vi "Tell Parent Inspect.vi"(4 "Msg":refnum<class "Msg.lvclass">, 6 "Within Unified Msgs":bool, 7 "Actor in":refnum<class "Actor.lvclass">, 8 "Error in":errorcluster) -> (0 "Error out":errorcluster, 2 "Proceed":bool=TRUE, 5 "Actor out":refnum<class "Actor.lvclass">)   [LabVIEW 2025, in "jettl.lvlib"]
uses:
  jettl.lvlib
  Actor/Actor.lvclass
  Msg/Msg.lvclass
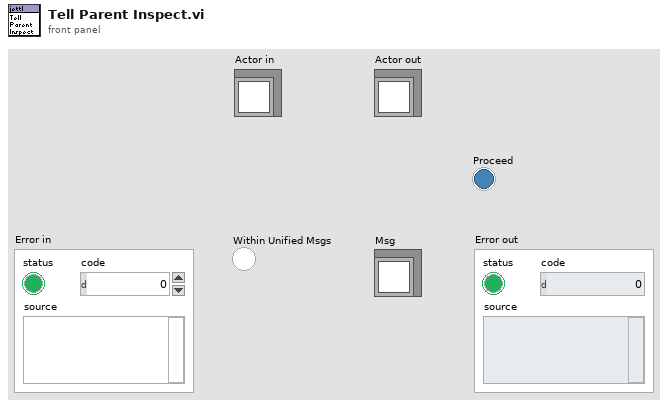
[diagram p1: front panel]
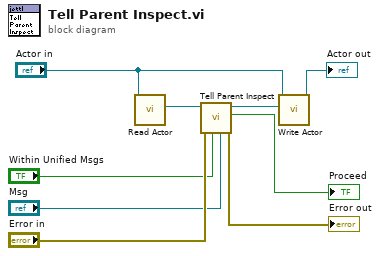
[diagram p0: block diagram]
diagram:
  n1 = call-dynamic "Read Actor.vi"("Actor in"="Actor in") -> ("Actor"=w7:refnum<class "Actor.lvclass">)  [unwired: 10 in]
  n2 = call-dynamic "Tell Parent Inspect.vi"("Msg"="Msg", "Within Unified Msgs"="Within Unified Msgs", "Error in"="Error in", "Actor in"=w7) -> ("Error out"=→"Error out":errorcluster, "Proceed"=→"Proceed":bool, "Actor out"=w6:refnum<class "Actor.lvclass">)  [unwired: 5 in]
  n3 = call-dynamic "Write Actor.vi"("Actor"=w6, "Actor in"="Actor in") -> ("Actor out"=→"Actor out":refnum<class "Actor.lvclass">)  [unwired: 9 in]
